vi "CRC8.vi"(11 "Data":u8[](array[numeric])) -> (3 "CRC8":u8=49)   [LabVIEW 2009]
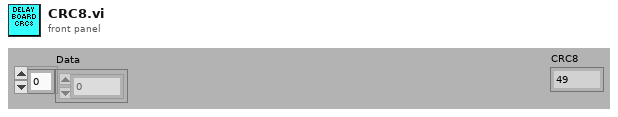
[diagram p1: front panel]
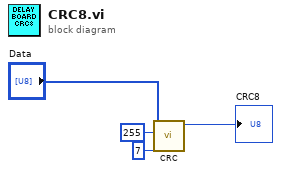
[diagram p0: block diagram]
diagram:
  n1 = call "CRC.vi"("Polynomial"=u8 7, "ResetValue"=u8 255, "Data"="Data") -> ("CRC8"=→"CRC8":u8)  [unwired: 8 in]
